vi "Construct TCP Client.vi"(9 "Local Port (0)":u16, 10 "Remote Port or Service Name":u16, 11 "Address":string) -> (3 "TCP Client out":refnum<class "TCP Client.lvclass">)   [LabVIEW 2017, in "TCP Interface.lvlib" / "TCP Client.lvclass"]
uses:
  <vilib>/gpm_packages/@cs/Network-sink/Source/TCP Interface/TCP Client/TCP Client.lvclass
  <vilib>/gpm_packages/@cs/Network-sink/Source/TCP Interface/TCP Client/TCP Client.lvclass/TCP Client.ctl
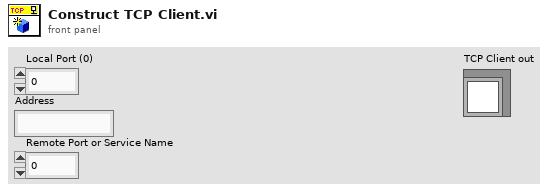
[diagram p1: front panel]
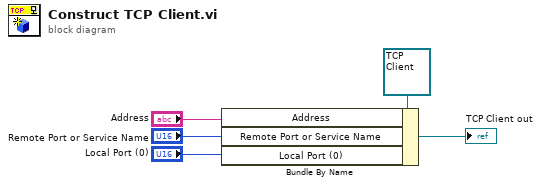
[diagram p0: block diagram]
diagram:
  n1 = Bundle By Name(cluster=refnum<class "TCP Client.lvclass"> refnum ("TCP Client in"), "Address"="Address", "Remote Port or Service Name"="Remote Port or Service Name", "Local Port (0)"="Local Port (0)") -> (→"TCP Client out":refnum<class "TCP Client.lvclass">)
